vi "Git History.vi"(7 "Git Type":T1, 8 "Error in":errorcluster caption="Error in (no error)", 10 "Branch Hierarchy":string[](array[string])=["master", "dev", "feature", "hot-fix"], 11 "Working Directory":path=path "C:/projects/DMC/Tooling/Git-Action-Service") -> (0 "Error out":errorcluster, 3 "File Change Map":T2 {"File Change Info"."Timestamp" format="%<%.0X %x>T"})   [LabVIEW 2023]
uses:
  <vilib>/DMC/VIDoc/Printers/Confluence/Confluence Printer/Types/File Change Map.ctl
  Git Type.ctl
  <vilib>/Hampel Software Engineering/Git API/Git API/GIT-api.lvclass/GIT-api.ctl
  <vilib>/Utility/miscctls.llb/LVMapReplaceAction.ctl
  647a7ef8-24e7-4281-b4f0-7b8b33f63b81.vi
  <vilib>/Utility/error.llb/Trim Whitespace One-Sided.vi
  <vilib>/Hampel Software Engineering/Git API/Git API/GIT-api.lvclass
  <vilib>/DMC/VIDoc/Printers/Confluence/Confluence Printer/VIDoc Printer - Confluence.lvclass
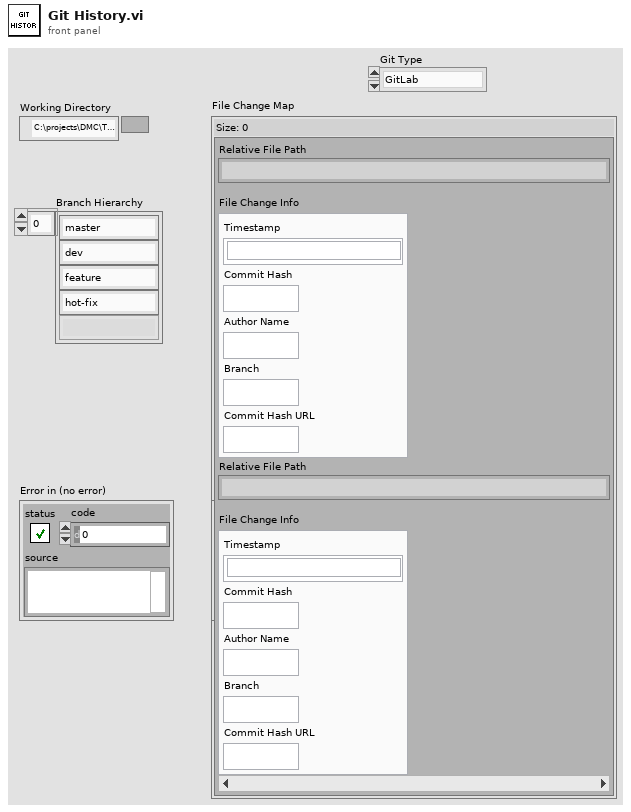
[diagram p1: front panel]
types:
  T1 = typedef "Git Type.ctl" = enum16{"GitLab", "GitHub", "BitBucket"}
  T2 = typedef "VIDoc Printer - Confluence.lvlib/VIDoc Printer - Confluence.lvclass/File Change Map.ctl" = map{string, cluster{"Timestamp":timestamp, "Commit Hash":string, "Author Name":string, "Branch":string, "Commit Hash URL":string}}
  T3 = typedef "LVMapReplaceAction.ctl" = enum32{"Modify Entry only if found", "Add or Modify Entry", "Delete Entry"}
  T4 = cluster{"Timestamp":timestamp, "Commit Hash":string, "Author Name":string, "Branch":string, "Commit Hash URL":string}
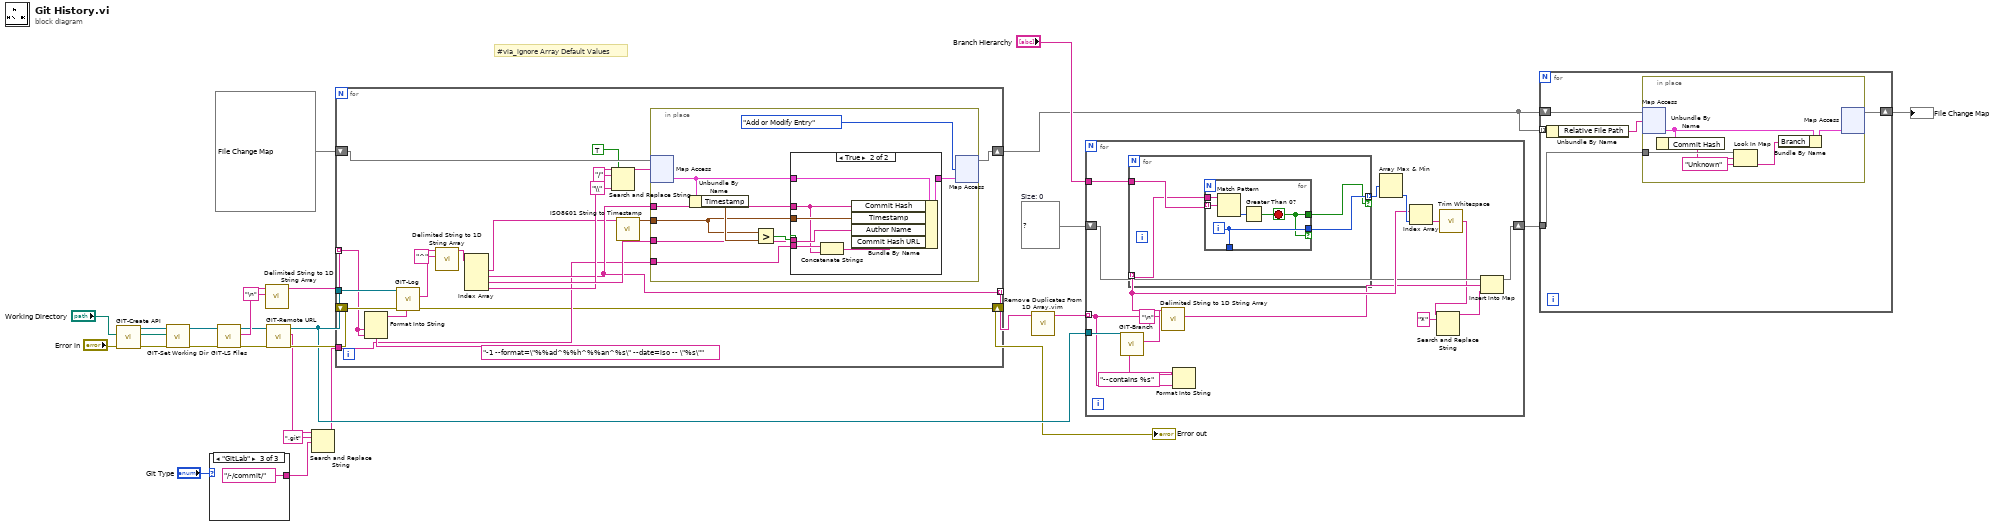
[diagram p0: block diagram]
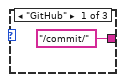
[diagram p2: hidden frame]
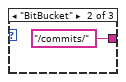
[diagram p3: hidden frame]
diagram:
  w13 = map{string, string} {}  # Size: 0
  # "#via_ignore Array Default Values"
  n1 = call <vilib>:"GIT-Create API.vi"("error in"="Error in") -> ("error out"=w26:errorcluster, "git-api out"=w27:refnum<class "GIT-api.lvclass">)  [unwired: 9 in]
  n2 = call <vilib>:"GIT-Set Working Dir.vi"("error in"=w26, "Working Directory"="Working Directory", "git-api in"=w27) -> ("error out"=w24:errorcluster, "git-api out"=w23:refnum<class "GIT-api.lvclass">)  [unwired: 7 in]
  n3 = case shown="\"GitLab\"" "Git Type" {
    tunnel: ["/commit/" "/commits/" "/-/commit/"] -> w3
    frame "GitHub" {
    }
    frame "BitBucket" {
    }
    frame "GitLab" {
    }
  }
  n4 = call <vilib>:"GIT-LS Files.vi"("error in"=w24, "git-api in"=w23) -> ("error out"=w10:errorcluster, "std out"=w22:string, "git-api out"=w9:refnum<class "GIT-api.lvclass">)  [unwired: 7 in]
  n5 = call <vilib>:"Delimited String to 1D String Array.vi"("delimiter"="\n", "delimited string"=w22) -> ("string array"=w19:string[])  [unwired: 9 in]
  n6 = call <vilib>:"GIT-Remote URL.vi"("error in"=w10, "git-api in"=w9) -> ("error out"=w8:errorcluster, "remote url"=w2:string, "git-api out"=w7:refnum<class "GIT-api.lvclass">)  [unwired: 7 in]
  n7 = Search and Replace String(input string=w2, search string=".git", replace string=w3) -> (result string=w1:string)  [unwired: 5 in, 3 out]
  n8 = for {
    shift-right: [w31] -> w6
    shift-left: w8 -> [w42]
    shift-right: [w50] -> w14
    shift-left: T2 {} ("File Change Map") -> [w51]
    tunnel: w19 -> [w36] mode=indexing
    tunnel: w7 -> [w43]
    tunnel: [w35] -> w17 mode=indexing
    tunnel: w1 -> [w34]
    n9 = Format Into String(format string="-1 --format=\"%%ad^%%h^%%an^%s\" --date=iso -- \"%s\"", w36, w36) -> (resulting string=w40:string)  [unwired: 2 in, 1 out]
    n10 = call <vilib>:"GIT-Log.vi"("param"=w40, "error in"=w42, "git-api in"=w43) -> ("error out"=w31:errorcluster, "std out"=w39:string)  [unwired: 6 in, 1 out]
    n11 = call <vilib>:"Delimited String to 1D String Array.vi"("delimiter"="^", "delimited string"=w39) -> ("string array"=w37:string[])  [unwired: 9 in]
    n12 = Index Array(array=w37) -> (element #1=w33:string, element #2=w35:string, element #3=w49:string, element #4=w47:string)  [unwired: 4 in]
    n13 = Search and Replace String(replace all?=TRUE ("replace all? (F)"), input string=w47, search string="/", replace string="\\" ("replace string (\"\")")) -> (result string=w48:string)  [unwired: 4 in, 3 out]
    n14 = call <vilib>:"ISO8601 String to Timestamp.vi"("ISO8601 String"=w33) -> ("Timestamp"=w32:timestamp)  [unwired: 8 in, 2 out]
    n15 = in-place {
      in-place-border: w32 -> [w55]
      in-place-border: w35 -> [w54]
      in-place-border: w49 -> [w53]
      in-place-border: w34 -> [w52]
      n16 = in-place-map #1(w51, w48) -> (w59:T4)  [unwired: 1 in, 1 out]
      n17 = Unbundle By Name(w59) -> ("Timestamp"=w57:timestamp)
      n18 = Greater?(x=w55, y=w57) -> (0:w56:bool)
      n19 = case shown="True" w56 {
        tunnel: w59 -> [w61 w68]
        tunnel: [w61 w67] -> w58
        tunnel: w55 -> [_ w66]
        tunnel: w54 -> [_ w63]
        tunnel: w53 -> [_ w65]
        tunnel: w52 -> [_ w64]
        frame False {
        }
        frame True {
          n20 = Concatenate Strings(w64, w63) -> (w62:string)
          n21 = Bundle By Name(cluster=w68, "Commit Hash"=w63, "Timestamp"=w66, "Author Name"=w65, "Commit Hash URL"=w62) -> (w67:T4)
        }
      }
      n22 = in-place-map #1(w58, LVMapReplaceAction."Add or Modify Entry" ("action")) -> (w50:T2)  [unwired: 2 out]
    }
  }
  "Error out" <- w6
  n23 = call "Remove Duplicates From 1D Array.vim"("array"=w17) -> ("array with duplicates removed"=w16:string[])  [unwired: 10 in]
  n24 = for {
    tunnel: w16 -> [w73] mode=indexing
    tunnel: w7 -> [w84]
    tunnel: "Branch Hierarchy" -> [w76]
    shift-right: [w74] -> w12
    shift-left: w13 -> [w75]
    n25 = Format Into String(format string="--contains %s", w73) -> (resulting string=w78:string)  [unwired: 2 in, 1 out]
    n26 = call <vilib>:"GIT-Branch.vi"("param"=w78, "git-api in"=w84) -> ("std out"=w80:string)  [unwired: 7 in, 2 out]
    n27 = call <vilib>:"Delimited String to 1D String Array.vi"("delimiter"="\n", "delimited string"=w80) -> ("string array"=w77:string[])  [unwired: 9 in]
    n28 = for {
      tunnel: w77 -> [w87] mode=indexing
      tunnel: [w86] -> w83 mode=indexing if=w85
      tunnel: w76 -> [w88]
      n29 = for {
        tunnel: w87 -> [w93]
        tunnel: w88 -> [w92] mode=indexing
        tunnel: [w89] -> w85
        tunnel: [w90] -> _
        tunnel: [w90] -> w86 if=w89
        i -> [w90]
        stop <- w89 stop-if-true
        n30 = Match Pattern(string=w93, regular expression=w92) -> (offset past match=w91:i32)  [unwired: 4 out]
        n31 = Greater Than 0?(x=w91) -> (x > 0?=w89:bool)
      }
    }
    n32 = Array Max & Min(array=w83) -> (min index (indices)=w81:i32)  [unwired: 3 out]
    n33 = Index Array(array=w77, index=w81) -> (element=w82:string)
    n34 = call <vilib>:"Trim Whitespace.vi"("string"=w82) -> ("trimmed string"=w72:string)  [unwired: 1 in]
    n35 = Search and Replace String(input string=w72, search string="*") -> (result string=w71:string)  [unwired: 6 in, 3 out]
    n36 = Insert Into Map(map in=w75, key=w73, value=w71) -> (map out=w74:map{string, string})  [unwired: 2 out]
  }
  n37 = for {
    shift-right: [w94] -> w11
    shift-left: w14 -> [w98]
    tunnel: w14 -> [w97] mode=indexing
    tunnel: w12 -> [w95]
    n38 = Unbundle By Name(w97) -> ("Relative File Path"=w96:string)
    n39 = in-place {
      in-place-border: w95 -> [w102]
      n40 = in-place-map #2(w98, w96) -> (w104:T4)  [unwired: 1 in, 1 out]
      n41 = Unbundle By Name(w104) -> ("Commit Hash"=w101:string)
      n42 = Look In Map(map=w102, key=w101, default value="Unknown") -> (value=w100:string)  [unwired: 1 out]
      n43 = Bundle By Name(cluster=w104, "Branch"=w100) -> (w103:T4)
      n44 = in-place-map #2(w103) -> (w94:T2)  [unwired: 1 in, 2 out]
    }
  }
  "File Change Map" <- w11
